vi "Pasco Auton Drive Shoot.vi"(8 "Encoder total":dbl, 9 "Array":i32, 10 "Power":dbl, 11 "time/distance":dbl) -> (0 "Encoder total":dbl, 1 "Array Out":i32, 2 "Power":dbl)   [LabVIEW 2011]
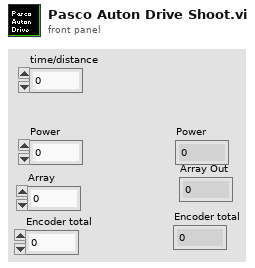
[diagram p1: front panel]
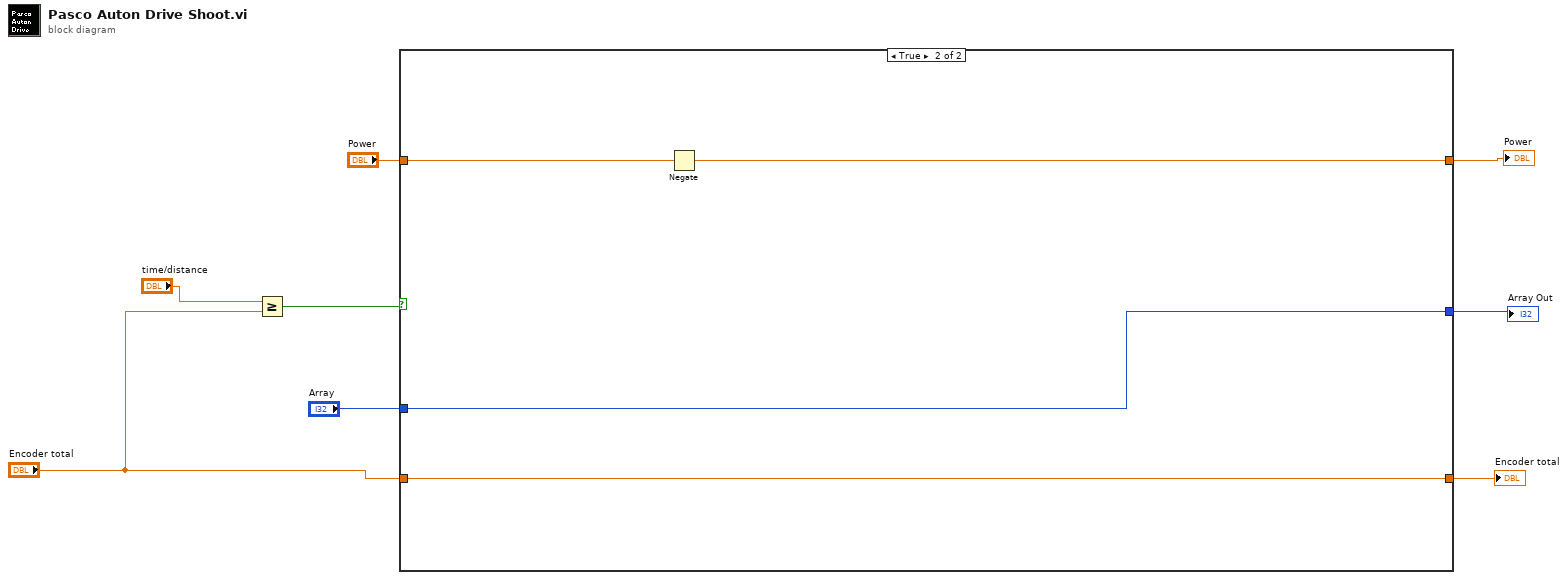
[diagram p0: block diagram]
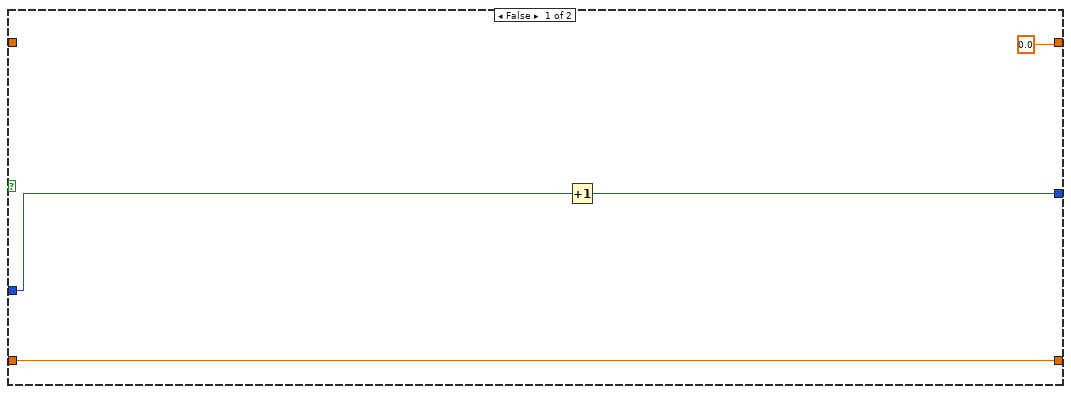
[diagram p2: hidden frame]
diagram:
  n1 = Greater Or Equal?(x="time/distance", y="Encoder total") -> (x >= y?=w1:bool)
  n2 = case shown="True" w1 {
    tunnel: [0.0 w13] -> w8
    tunnel: [w10 w15] -> w7
    tunnel: [w12 w16] -> w6
    tunnel: "Array" -> [w9 w15]
    tunnel: "Encoder total" -> [w12 w16]
    tunnel: "Power" -> [_ w14]
    frame False {
      n3 = Increment(x=w9) -> (x+1=w10:i32)
    }
    frame True {
      n4 = Negate(x=w14) -> (-x=w13:dbl)
    }
  }
  "Power" <- w8
  "Array Out" <- w7
  "Encoder total" <- w6
